vi "GOLPI full test - part test vector double.vi"(6 "column vector?":bool, 7 "set: use temporary file?":bool, 8 "error in (no error)":errorcluster, 9 "test value":dbl[](array[numeric])=[1.234, 2.345, 3.456], 10 "variable name in":string, 11 "GOLPI ref. in":T1={"pipe handle"={"lv_proc.dll file path"=path "", "process instance handle"=[], "debug mode"=FALSE, "debug data"=[]}, "fast read timeout [ms]"=0, "fast read settle time [ms]"=0, "fast read to multiple [ms]"=0, "max elements per input line"=0, "slow read timeout [ms]"=5000, "stdin double format specifier"="%_16e", "max elements per stdout output column"=100, "console mode bitstream"=FALSE, "bitstream first read timeout [ms]"=1000, "bitstream read timeout [ms]"=50, "struct transfer possible"=FALSE, "matlab mode"=FALSE}) -> (0 "error out":errorcluster, 2 "test result":bool, 3 "GOLPI ref. out":T1={"pipe handle"={"lv_proc.dll file path"=path "", "process instance handle"=[], "debug mode"=FALSE, "debug data"=[]}, "fast read timeout [ms]"=0, "fast read settle time [ms]"=0, "fast read to multiple [ms]"=0, "max elements per input line"=0, "slow read timeout [ms]"=5000, "stdin double format specifier"="%_16e", "max elements per stdout output column"=100, "console mode bitstream"=FALSE, "bitstream first read timeout [ms]"=1000, "bitstream read timeout [ms]"=50, "struct transfer possible"=FALSE, "matlab mode"=FALSE})   [LabVIEW 2020, in "GOLPI library.lvlib"]
doc: "part of GOLPI full test.vi - checks vectors"
uses:
  GOLPI library.lvlib
  GOLPI reference Type Def.ctl
  Pipe Handle.ctl
  Set 1D Array Double.vi
  Get 1D Array Double.vi
  LV Process library.lvlib
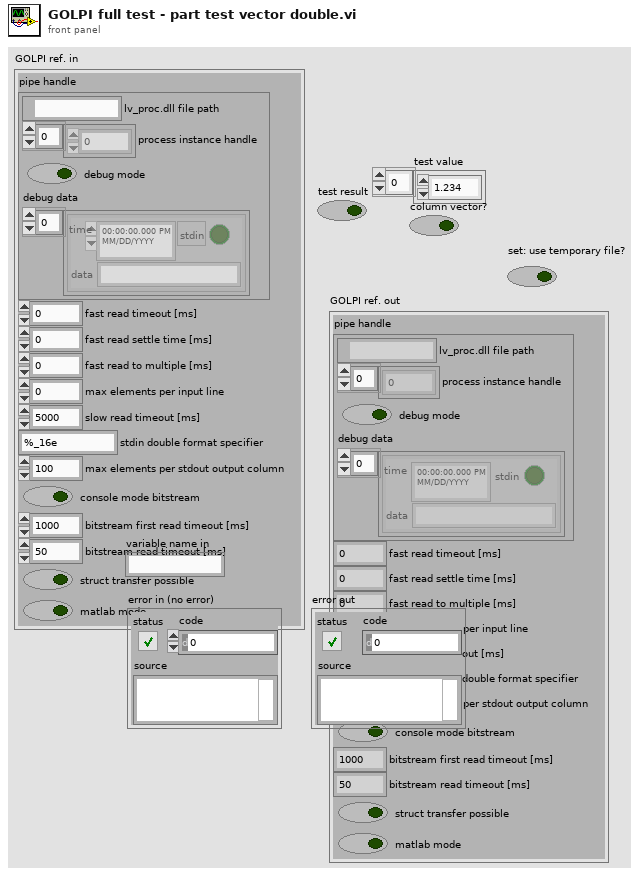
[diagram p1: front panel]
types:
  T1 = typedef "GOLPI library.lvlib/GOLPI reference Type Def.ctl" = cluster{"pipe handle":T2, "fast read timeout [ms]":u32, "fast read settle time [ms]":u32, "fast read to multiple [ms]":u32, "max elements per input line":u32, "slow read timeout [ms]":u32, "stdin double format specifier":string, "max elements per stdout output column":u32, "console mode bitstream":bool, "bitstream first read timeout [ms]":u32, "bitstream read timeout [ms]":u32, "struct transfer possible":bool, "matlab mode":bool}
  T2 = typedef "LV Process library.lvlib/Pipe Handle.ctl" = cluster{"lv_proc.dll file path":path, "process instance handle":u32[], "debug mode":bool, "debug data":cluster{"time":timestamp, "stdin":bool, "data":string}[]}
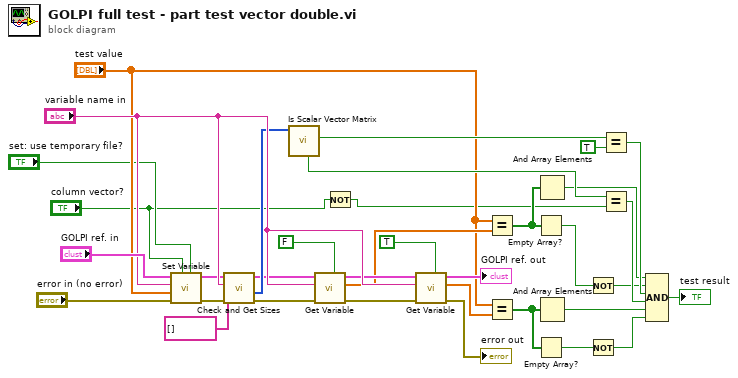
[diagram p0: block diagram]
diagram:
  n1 = call-poly "Set Variable.vi"("use temporary file? (F)"="set: use temporary file?", "column vector?"="column vector?", "error in"="error in (no error)", "value"="test value", "variable name"="variable name in", "GOLPI ref. in"="GOLPI ref. in") -> ("error out"=w11:errorcluster, "GOLPI ref. out"=w12:T1)  [unwired: 4 in]
  n2 = call "Check and Get Sizes.vi"("error in (no error)"=w11, "test commands"=string[] [], "variable name"="variable name in", "GOLPI ref. in"=w12) -> ("error out"=w14:errorcluster, "octave sizes"=w15:i32[], "GOLPI ref. out"=w13:T1)  [unwired: 4 in, 1 out]
  n3 = call "Is Scalar Vector Matrix.vi"("octave sizes"=w15) -> ("is vector?"=w19:bool, "row vector?"=w16:bool)  [unwired: 5 in, 4 out]
  n4 = call-poly "Get Variable.vi"("use temporary file? (F)"=FALSE ("use temporary file?"), "error in"=w14, "variable name"="variable name in", "GOLPI ref. in"=w13) -> ("error out"=w22:errorcluster, "value"=w10:dbl[], "GOLPI ref. out"=w21:T1)  [unwired: 5 in]
  n5 = Not(x="column vector?") -> (.not. x?=w2:bool)
  n6 = call-poly "Get Variable.vi"("use temporary file? (F)"=TRUE ("use temporary file?"), "error in"=w22, "variable name"="variable name in", "GOLPI ref. in"=w21) -> ("error out"=→"error out":errorcluster, "value"=w27:dbl[], "GOLPI ref. out"=→"GOLPI ref. out":T1)  [unwired: 5 in]
  n7 = Equal?(x="test value", y=w10) -> (x = y?=w9:bool[])
  n8 = Equal?(x="test value", y=w27) -> (x = y?=w25:bool[])
  n9 = Empty Array?(array=w9) -> (empty?=w8:bool)
  n10 = Empty Array?(array=w25) -> (empty?=w26:bool)
  n11 = And Array Elements(Boolean array=w9) -> (logical AND=w6:bool)
  n12 = And Array Elements(Boolean array=w25) -> (logical AND=w28:bool)
  n13 = Not(x=w8) -> (.not. x?=w7:bool)
  n14 = Not(x=w26) -> (.not. x?=w29:bool)
  n15 = Equal?(x=w19, y=TRUE) -> (x = y?=w20:bool)
  n16 = Equal?(x=w16, y=w2) -> (x = y?=w17:bool)
  n17 = Compound Arithmetic op=AND(w6, w7, w20, w17, w28, w29) -> (→"test result":bool)
